vi "Set Message Field Representation.vi"(8 "error in (no error)":errorcluster, 10 "MessageElementType":T1, 11 "Control ref in":refnum<vi>) -> (0 "error out":errorcluster, 3 "Control ref out":refnum<vi>)   [LabVIEW 2019, in "gRPC Scripting Tools.lvlib"]
uses:
  gRPC Scripting Tools.lvlib
  <vilib>/numeric/LVNumericRepresentation.ctl
  TypeDefs/Message Element Type.ctl
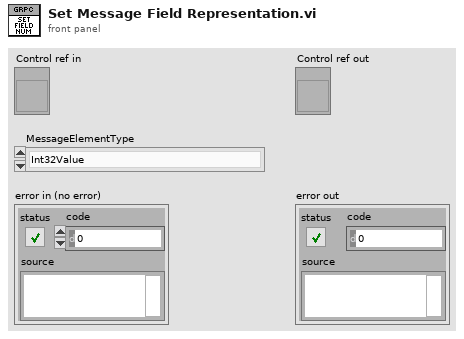
[diagram p1: front panel]
types:
  T1 = typedef "gRPC Scripting Tools.lvlib/Message Element Type.ctl" = enum32{"Int32Value", "FloatValue", "DoubleValue", "BoolValue", "StringValue", "MessageValue", "Int64Value", "UInt32Value", "UInt64Value", "EnumValue"}
  T2 = typedef "LVNumericRepresentation.ctl" = enum32{"Extended Precision", "Double Precision", "Single Precision", "Long", "Word", "Byte", "Unsigned Long", "Unsigned Word", "Unsigned Byte", "Complex Extended", "Complex Double", "Complex Single", "Quad", "Unsigned Quad", "Fixed-Point"}
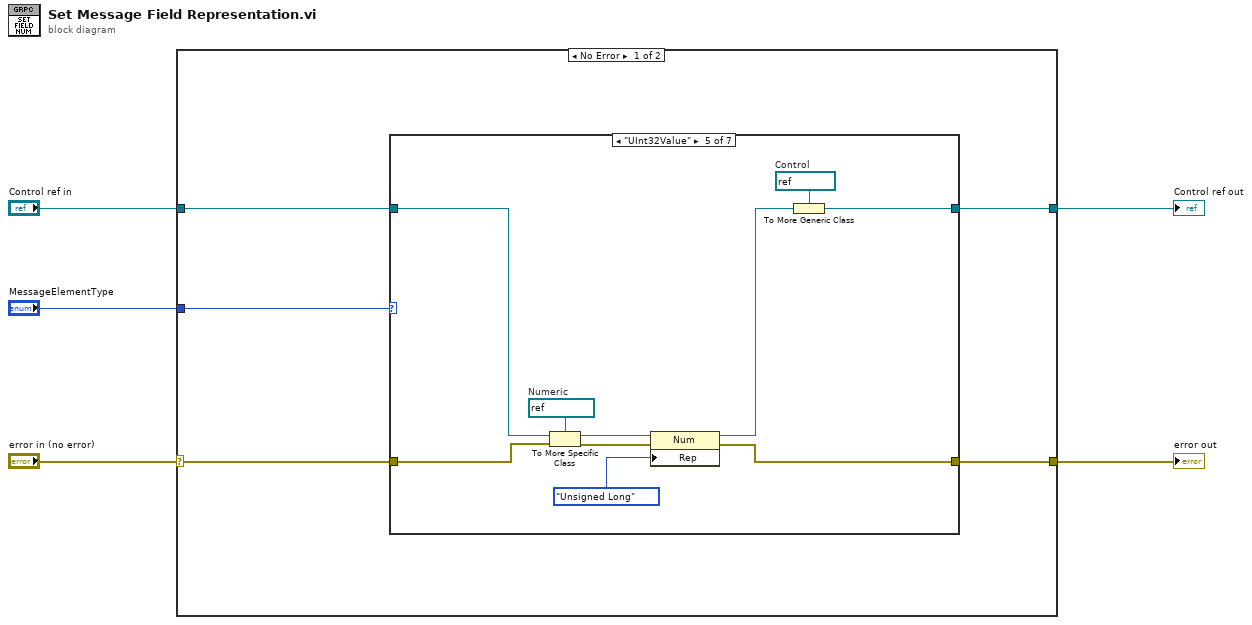
[diagram p0: block diagram]
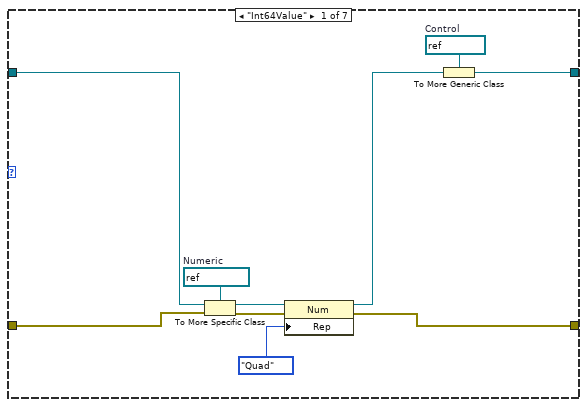
[diagram p2: hidden frame]
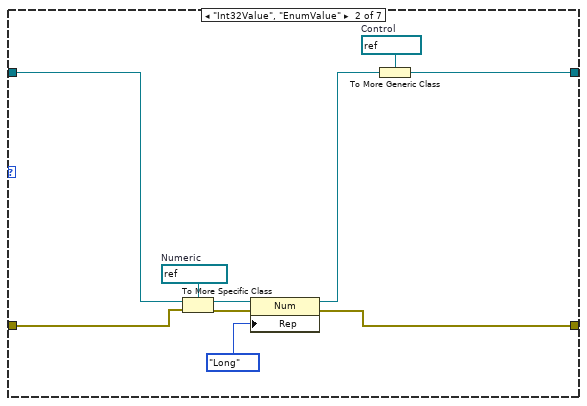
[diagram p3: hidden frame]
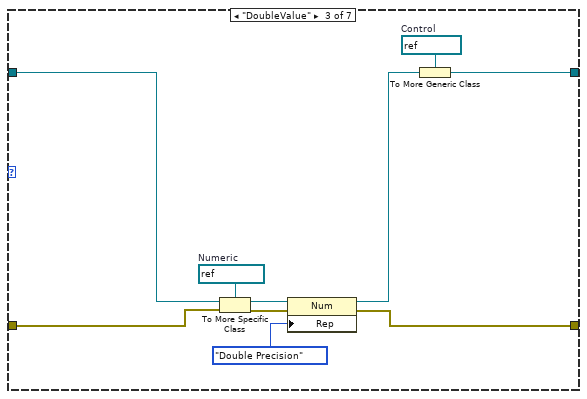
[diagram p4: hidden frame]
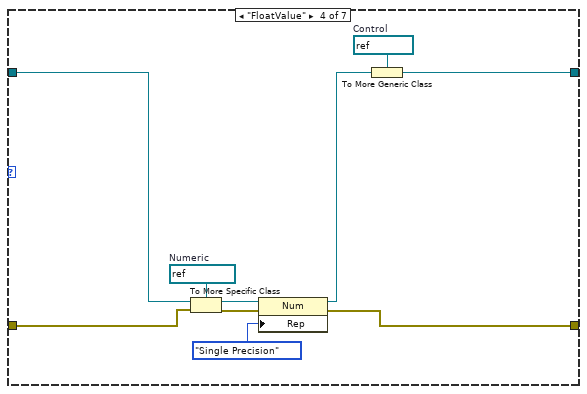
[diagram p5: hidden frame]
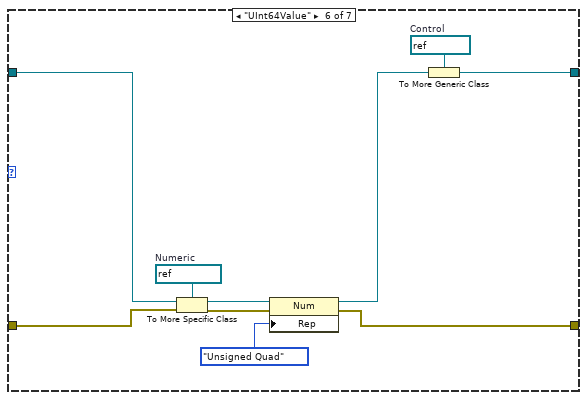
[diagram p6: hidden frame]
diagram:
  n1 = case shown="No Error" "error in (no error)" {
    selector: "error in (no error)" -> [w6 w73]
    tunnel: [w10 w74] -> w5
    tunnel: "MessageElementType" -> [w9 _]
    tunnel: [w8 w73] -> w3
    tunnel: "Control ref in" -> [w7 w74]
    frame No Error {
      n2 = case shown="\"UInt32Value\"" w9 {
        tunnel: w7 -> [w13 w30 w40 w50 w54 w64 w72]
        tunnel: w6 -> [w14 w28 w38 w48 w53 w63 w71]
        tunnel: [w12 w24 w34 w44 w51 w61 w71] -> w8
        tunnel: [w11 w21 w31 w41 w52 w62 w72] -> w10
        frame "Int64Value" {
          w16 = refnum<vi> refnum  # Control
          w20 = refnum<vi> refnum  # Numeric
          n3 = To More Specific Class(target class=w20, reference=w13, error in=w14) -> (specific class reference=w19:refnum<vi>, error out=w18:errorcluster)
          n4 = property class="Num"(reference=w19, error in=w18, "Rep"=LVNumericRepresentation."Quad" ("Representation")) -> (reference out=w15:refnum<vi>, error out=w12:errorcluster)
          n5 = To More Generic Class(target class=w16, reference=w15) -> (generic class reference=w11:refnum<vi>)
        }
        frame "Int32Value", "EnumValue" {
          w23 = refnum<vi> refnum  # Control
          w29 = refnum<vi> refnum  # Numeric
          n6 = To More Specific Class(target class=w29, reference=w30, error in=w28) -> (specific class reference=w27:refnum<vi>, error out=w26:errorcluster)
          n7 = property class="Num"(reference=w27, error in=w26, "Rep"=LVNumericRepresentation."Long" ("Representation")) -> (reference out=w22:refnum<vi>, error out=w24:errorcluster)
          n8 = To More Generic Class(target class=w23, reference=w22) -> (generic class reference=w21:refnum<vi>)
        }
        frame "DoubleValue" {
          w33 = refnum<vi> refnum  # Control
          w39 = refnum<vi> refnum  # Numeric
          n9 = To More Specific Class(target class=w39, reference=w40, error in=w38) -> (specific class reference=w37:refnum<vi>, error out=w36:errorcluster)
          n10 = property class="Num"(reference=w37, error in=w36, "Rep"=LVNumericRepresentation."Double Precision" ("Representation")) -> (reference out=w32:refnum<vi>, error out=w34:errorcluster)
          n11 = To More Generic Class(target class=w33, reference=w32) -> (generic class reference=w31:refnum<vi>)
        }
        frame "FloatValue" {
          w43 = refnum<vi> refnum  # Control
          w49 = refnum<vi> refnum  # Numeric
          n12 = To More Specific Class(target class=w49, reference=w50, error in=w48) -> (specific class reference=w47:refnum<vi>, error out=w46:errorcluster)
          n13 = property class="Num"(reference=w47, error in=w46, "Rep"=LVNumericRepresentation."Single Precision" ("Representation")) -> (reference out=w42:refnum<vi>, error out=w44:errorcluster)
          n14 = To More Generic Class(target class=w43, reference=w42) -> (generic class reference=w41:refnum<vi>)
        }
        frame "UInt32Value" {
          w56 = refnum<vi> refnum  # Control
          w60 = refnum<vi> refnum  # Numeric
          n15 = To More Specific Class(target class=w60, reference=w54, error in=w53) -> (specific class reference=w59:refnum<vi>, error out=w58:errorcluster)
          n16 = property class="Num"(reference=w59, error in=w58, "Rep"=LVNumericRepresentation."Unsigned Long" ("Representation")) -> (reference out=w55:refnum<vi>, error out=w51:errorcluster)
          n17 = To More Generic Class(target class=w56, reference=w55) -> (generic class reference=w52:refnum<vi>)
        }
        frame "UInt64Value" {
          w66 = refnum<vi> refnum  # Control
          w70 = refnum<vi> refnum  # Numeric
          n18 = To More Specific Class(target class=w70, reference=w64, error in=w63) -> (specific class reference=w69:refnum<vi>, error out=w68:errorcluster)
          n19 = property class="Num"(reference=w69, error in=w68, "Rep"=LVNumericRepresentation."Unsigned Quad" ("Representation")) -> (reference out=w65:refnum<vi>, error out=w61:errorcluster)
          n20 = To More Generic Class(target class=w66, reference=w65) -> (generic class reference=w62:refnum<vi>)
        }
        frame "StringValue", Default {
        }
      }
    }
    frame Error {
    }
  }
  "Control ref out" <- w5
  "error out" <- w3
